vi "Cannon Projectile Game.vi"() -> ()   [LabVIEW 2012]
panel:
  out "Distance":dbl
  out "?":cluster{dbl[], dbl[]}(graph)
  out "Score":dbl
  out "Attempt":i32
  out "Wind (mph)":dbl
  out "Target Distance (m)":dbl
  in  "?":bool
  in  "?":bool
  in  "Height (m)":dbl
  in  "Power":dbl
  in  "Angle (deg)":dbl
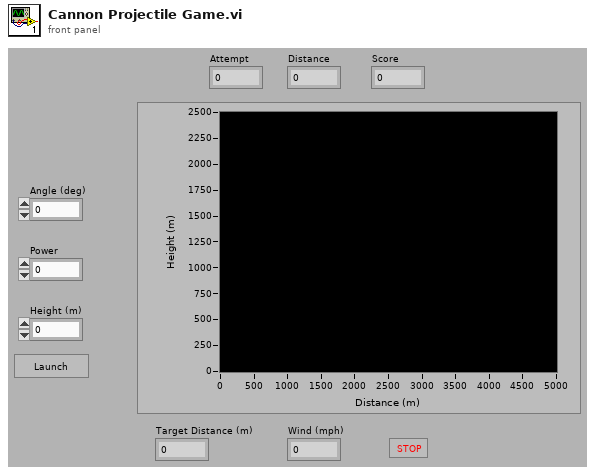
[diagram p1: front panel]
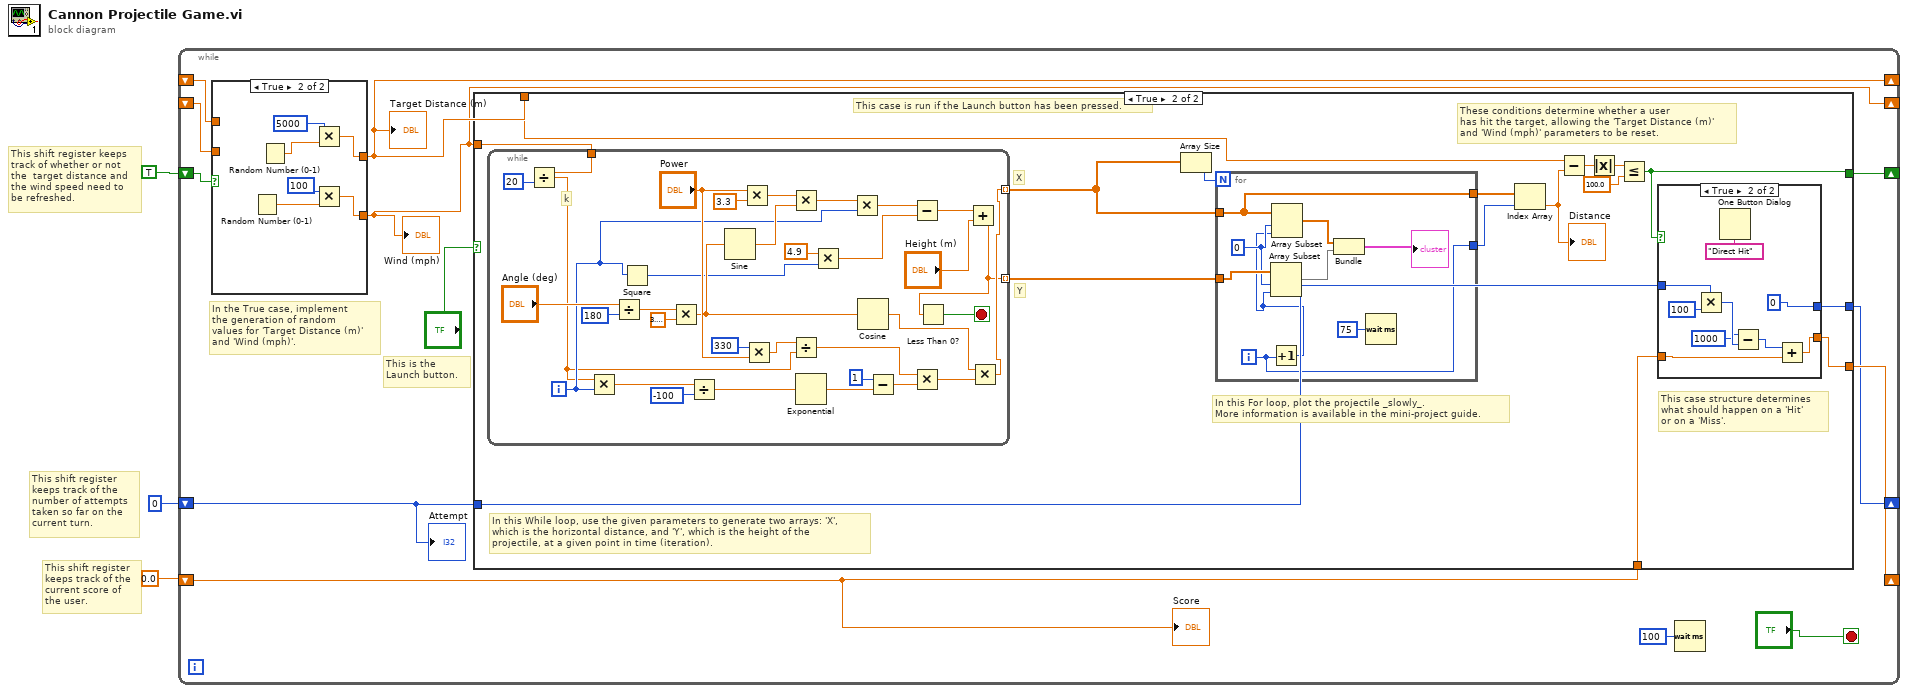
[diagram p0: block diagram]
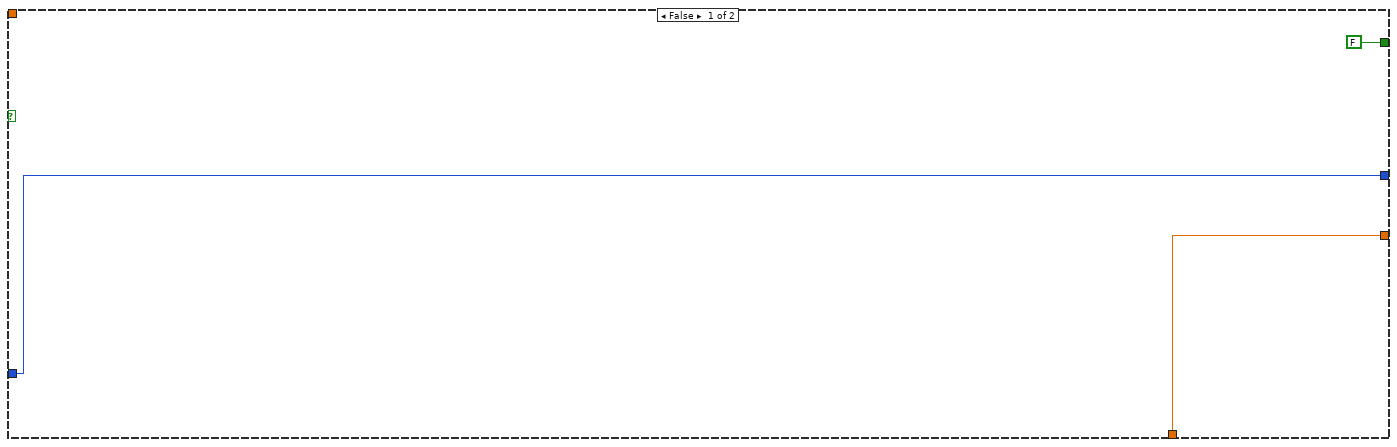
[diagram p3: hidden frame]
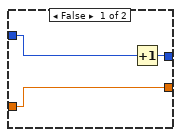
[diagram p4: hidden frame]
diagram:
  # "This shift register keeps\ntrack of whether or not\nthe  target distance and\nthe wind speed need to\nbe refreshed."
  # "This shift register\nkeeps track of the\ncurrent score of\nthe user."
  # "This shift register\nkeeps track of the\nnumber of attempts\ntaken so far on the\ncurrent turn."
  n1 = while {
    shift-right: [w14] -> _
    shift-left: 0.0 -> [w13]
    shift-right: [w12] -> _
    shift-left: 0 -> [w11]
    shift-right: [w9] -> _
    shift-left: TRUE -> [w8]
    shift-right: [w5] -> _
    shift-left: _ -> [w7]
    shift-right: [w4] -> _
    shift-left: _ -> [w6]
    stop <- "?" stop-if-true
    # "This is the Launch button."
    # "In the True case, implement\nthe generation of random\nvalues for 'Target Distance (m)'\nand 'Wind (mph)'."
    n2 = case shown="True" w8 {
      tunnel: [w18 w21] -> w5
      tunnel: [w17 w19] -> w4
      tunnel: w7 -> [w18 _]
      tunnel: w6 -> [w17 _]
      frame False {
      }
      frame True {
        n3 = Random Number (0-1)() -> (number: 0 to 1=w20:dbl)
        n4 = Random Number (0-1)() -> (number: 0 to 1=w22:dbl)
        n5 = Multiply(x=5000, y=w22) -> (x*y=w21:dbl)
        n6 = Multiply(x=100, y=w20) -> (x*y=w19:dbl)
      }
    }
    "Target Distance (m)" <- w5
    "Wind (mph)" <- w4
    n7 = case shown="True" "?" {
      tunnel: w5 -> [_ w42]
      tunnel: w4 -> [_ w43]
      tunnel: [w27 w38] -> w12
      tunnel: w11 -> [w27 w30]
      tunnel: [w26 w32] -> w14
      tunnel: w13 -> [w26 w31]
      tunnel: [FALSE w29] -> w9
      frame False {
      }
      frame True {
        # "X"
        # "Y"
        # "These conditions determine whether a user\nhas hit the target, allowing the 'Target Distance (m)'\nand 'Wind (mph)' parameters to be reset."
        # "This case is run if the Launch button has been pressed."
        # "This case structure determines\nwhat should happen on a 'Hit'\nor on a 'Miss'."
        # "In this For loop, plot the projectile _slowly_.\nMore information is available in the mini-project guide."
        # "In this While loop, use the given parameters to generate two arrays: 'X',\nwhich is the horizontal distance, and 'Y', which is the height of the\nprojectile, at a given point in time (iteration)."
        n8 = while {
          tunnel: w43 -> [w94]
          tunnel: [w85] -> w28 mode=indexing
          tunnel: [w65] -> w37 mode=indexing
          i -> [w68]
          stop <- w98 stop-if-true
          # "k"
          n9 = Divide(x=w94, y=20) -> (x/y=w66:dbl)
          n10 = Multiply(x=w66, y=w68) -> (x*y=w90:dbl)
          n11 = Divide(x="Angle (deg)", y=180) -> (x/y=w97:dbl)
          n12 = Square(x=w68) -> (x^2=w69:i32)
          n13 = Multiply(x=w97, y=3.141592653589793) -> (x*y=w80:dbl)
          n14 = Divide(x=w90, y=-100) -> (x/y=w88:dbl)
          n15 = Sine(x=w80) -> (sin(x)=w79:dbl)
          n16 = Multiply(x="Power", y=3.3) -> (x*y=w78:dbl)
          n17 = Multiply(x=330, y="Power") -> (x*y=w67:dbl)
          n18 = Multiply(x=w78, y=w79) -> (x*y=w77:dbl)
          n19 = Divide(x=w67, y=w66) -> (x/y=w92:dbl)
          n20 = Exponential(1:w88) -> (0:w84:dbl)
          n21 = Multiply(x=4.9, y=w69) -> (x*y=w70:dbl)
          n22 = Multiply(x=w77, y=w68) -> (x*y=w75:dbl)
          n23 = Cosine(x=w80) -> (cos(x)=w87:dbl)
          n24 = Subtract(x=1, y=w84) -> (x-y=w91:dbl)
          n25 = Subtract(x=w75, y=w70) -> (x-y=w74:dbl)
          n26 = Multiply(x=w92, y=w91) -> (x*y=w86:dbl)
          n27 = Add(x=w74, y="Height (m)") -> (x+y=w65:dbl)
          n28 = Less Than 0?(x=w65) -> (x < 0?=w98:bool)
          n29 = Multiply(x=w87, y=w86) -> (x*y=w85:dbl)
        }
        n30 = Array Size(array=w28) -> (size(s)=w33:i32)
        n31 = for {
          N: w33 -> [_]
          tunnel: w28 -> [w45]
          tunnel: w37 -> [w50]
          tunnel: [w45] -> w36
          tunnel: [w46] -> w35
          i -> [w46]
          w47 = u32 0 ("milliseconds to wait")
          n32 = Increment(x=w46) -> (x+1=w44:i32)
          n33 = Array Subset(array=w50, index=w47, length=w44) -> (w52:dbl[])
          n34 = Array Subset(array=w45, index=w47, length=w44) -> (w49:dbl[])
          n35 = Bundle(w49, w52) -> (→"?":cluster{dbl[], dbl[]})  [unwired: 1 out]
          n36 = Wait (ms)(milliseconds to wait=u32 75) -> ()  [unwired: 1 out]
        }
        n37 = Index Array(array=w36, index=w35) -> (element=w34:dbl)
        "Distance" <- w34
        n38 = Subtract(x=w42, y=w34) -> (x-y=w41:dbl)
        n39 = Absolute Value(x=w41) -> (abs(x)=w40:dbl)
        n40 = Less Or Equal?(x=w40, y=100.0) -> (x <= y?=w29:bool)
        n41 = case shown="True" w29 {
          tunnel: [w54 0] -> w38
          tunnel: w30 -> [w55 w63]
          tunnel: [w53 w62] -> w32
          tunnel: w31 -> [w53 w64]
          frame False {
            n42 = Increment(x=w55) -> (x+1=w54:i32)
          }
          frame True {
            n43 = Multiply(x=w63, y=100) -> (x*y=w59:i32)
            n44 = One Button Dialog(message="Direct Hit") -> ()  [unwired: 1 in, 1 out]
            n45 = Subtract(x=1000, y=w59) -> (x-y=w60:i32)
            n46 = Add(x=w60, y=w64) -> (x+y=w62:dbl)
          }
        }
      }
    }
    n47 = Wait (ms)(milliseconds to wait=u32 100) -> ()  [unwired: 1 out]
    "Score" <- w13
    "Attempt" <- w11
  }
